vi "Add User Code Library to Project.vi"(8 "error in (no error)":errorcluster, 10 "Project Path":path, 11 "Application reference":refnum<vi>) -> (0 "error out":errorcluster, 2 "User Code Server Library out":refnum<vi>)   [LabVIEW 2019, in "gRPC Template Creation Utility.lvlib"]
uses:
  gRPC Template Creation Utility.lvlib
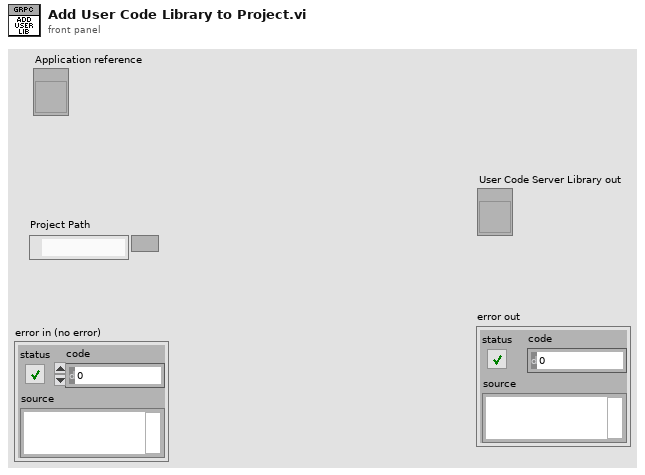
[diagram p1: front panel]
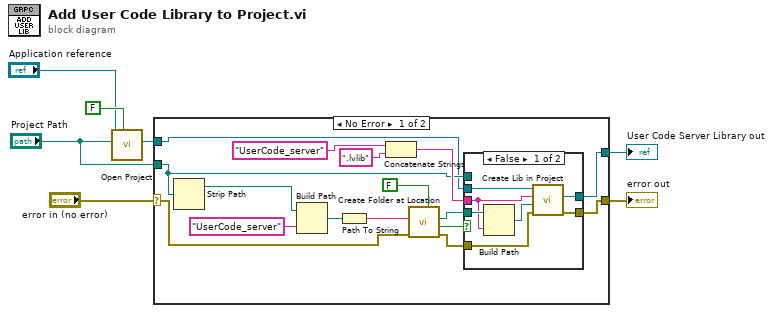
[diagram p0: block diagram]
diagram:
  n1 = call "Open Project.vi"("Open Project Window ?"=FALSE, "Project Path in"="Project Path", "Application reference"="Application reference") -> ("Project out"=w2:refnum<vi>)  [unwired: 6 in, 2 out]
  n2 = case shown="No Error" "error in (no error)" {
    selector: "error in (no error)" -> [w17 w32]
    tunnel: "Project Path" -> [w11 _]
    tunnel: [w16 w32] -> w6
    tunnel: [w9 _] -> w5
    tunnel: w2 -> [w8 _]
    frame No Error {
      n3 = Strip Path(path=w11) -> (stripped path=w21:path)  [unwired: 1 out]
      n4 = Build Path(base path=w21, name or relative path="UserCode_server") -> (appended path=w19:path)
      n5 = Path To String(path=w19) -> (string=w18:string)
      n6 = Concatenate Strings("UserCode_server", ".lvlib" ("string")) -> (w12:string)
      n7 = call "Create Folder at Location.vi"("Override existing (F)"=FALSE, "Error In"=w17, "Path"=w18) -> ("Error Out"=w15:errorcluster, "Already Exists ?"=w22:bool, "Full path out"=w10:path)  [unwired: 6 in]
      n8 = case shown="False" w22 {
        tunnel: [w30 w31] -> w16
        tunnel: w15 -> [w29 w31]
        tunnel: w12 -> [w27 _]
        tunnel: w11 -> [_ _]
        tunnel: w10 -> [w28 _]
        tunnel: [w25 _] -> w9
        tunnel: w8 -> [w24 _]
        frame False {
          n9 = Build Path(base path=w28, name or relative path=w27) -> (appended path=w26:path)
          n10 = call "Create Lib in Project.vi"("error in (no error)"=w29, "Save Path"=w26, "Library Name"=w27, "Project in"=w24) -> ("error out"=w30:errorcluster, "Library out"=w25:refnum<vi>)  [unwired: 5 in, 1 out]
        }
        frame True {
        }
      }
    }
    frame Error {
    }
  }
  "error out" <- w6
  "User Code Server Library out" <- w5
